vi "Start Acquisition.vi"(8 "error in (no error)":errorcluster, 10 "Period [ms]":i32, 11 "DAQ AI in":refnum<class "DAQ AI.lvclass">) -> (0 "error out":errorcluster, 3 "DAQ AI out":refnum<class "DAQ AI.lvclass">)   [LabVIEW 2020, in "DAQ AI.lvlib" / "DAQ AI.lvclass"]
uses:
  DAQ AI.lvclass
  DAQ AI Messages/Acquire Waveform Msg/Acquire Waveform Msg.lvclass
  C:/Program Files (x86)/National Instruments/LabVIEW 2026/vi.lib/ActorFramework/Message/Message.lvclass
  DAQ AI.lvclass/DAQ AI.ctl
  <vilib>/ActorFramework/Actor Framework.lvlib
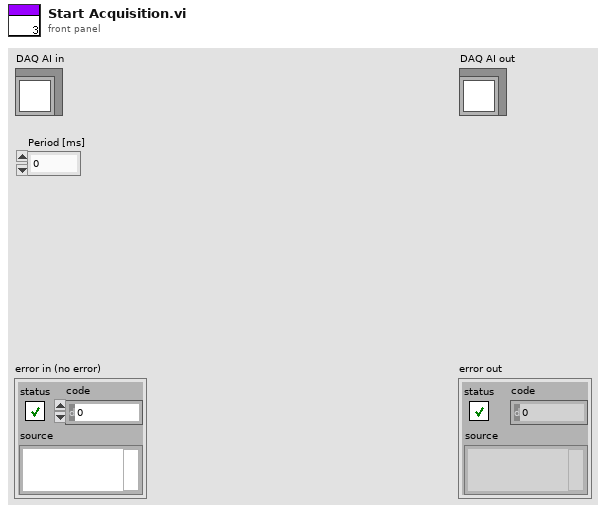
[diagram p1: front panel]
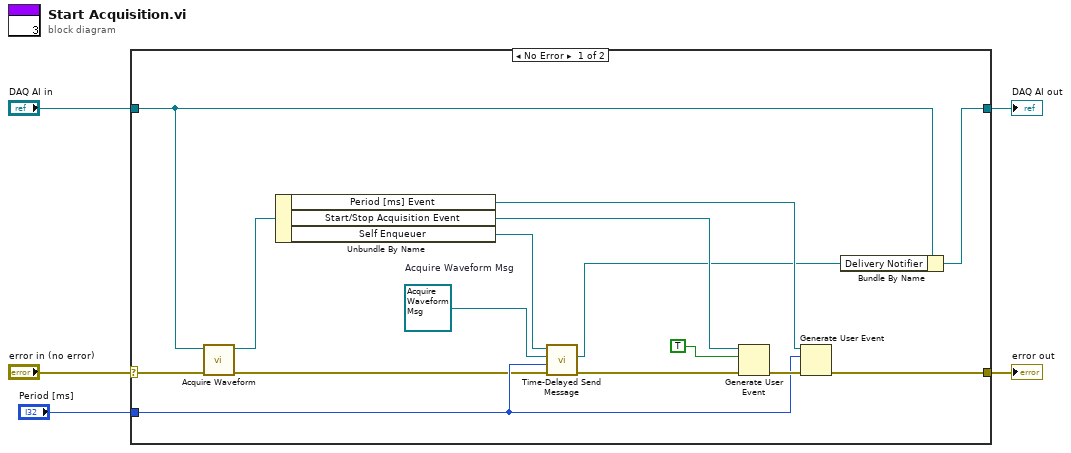
[diagram p0: block diagram]
diagram:
  n1 = case shown="No Error" "error in (no error)" {
    selector: "error in (no error)" -> [w8 w22]
    tunnel: [w16 w22] -> w4
    tunnel: [w11 w21] -> w2
    tunnel: "DAQ AI in" -> [w9 w21]
    tunnel: "Period [ms]" -> [w13 _]
    frame No Error {
      w14 = refnum<class "Acquire Waveform Msg.lvclass"> refnum  # Acquire Waveform Msg
      n2 = call "Acquire Waveform.vi"("error in (no error)"=w8, "DAQ AI in"=w9) -> ("error out"=w7:errorcluster, "DAQ AI out"=w6:refnum<class "DAQ AI.lvclass">)  [unwired: 8 in]
      n3 = Unbundle By Name(w6) -> ("Period [ms] Event"=w18:refnum<user-event>, "Start/Stop Acquisition Event"=w20:refnum<user-event>, "Self Enqueuer"=w15:refnum<class "Message Enqueuer.lvclass">)
      n4 = call <vilib>:"Time-Delayed Send Message.vi"("error in (no error)"=w7, "Milliseconds To Wait"=w13, "Message"=w14, "Message Enqueuer"=w15) -> ("error out"=w12:errorcluster, "Delivery Notifier"=w10:refnum<notifier>)  [unwired: 6 in]
      n5 = Generate User Event(user event=w20, event data cluster=TRUE ("event data"), error in=w12) -> (error out=w17:errorcluster)  [unwired: 1 in, 1 out]
      n6 = Generate User Event(user event=w18, event data cluster=w13, error in=w17) -> (error out=w16:errorcluster)  [unwired: 1 in, 1 out]
      n7 = Bundle By Name(cluster=w9, "Delivery Notifier"=w10) -> (w11:refnum<class "DAQ AI.lvclass">)
    }
    frame Error {
    }
  }
  "error out" <- w4
  "DAQ AI out" <- w2
